vi "Top Level.vi"() -> ()   [LabVIEW 2018]
panel:
  in  "Frame Control":enum32{"0", "1", "2", "3", "4", "5", "6"}(tab)
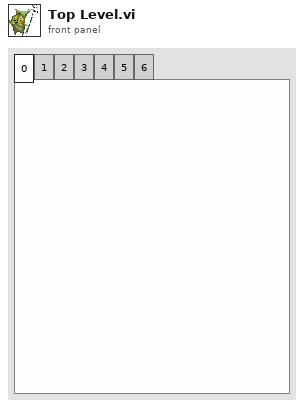
[diagram p1: front panel]
types:
  T1 = enum16{"Get_Item", "Yahaha!", "Korok_Pop", "Korok_Solve"}
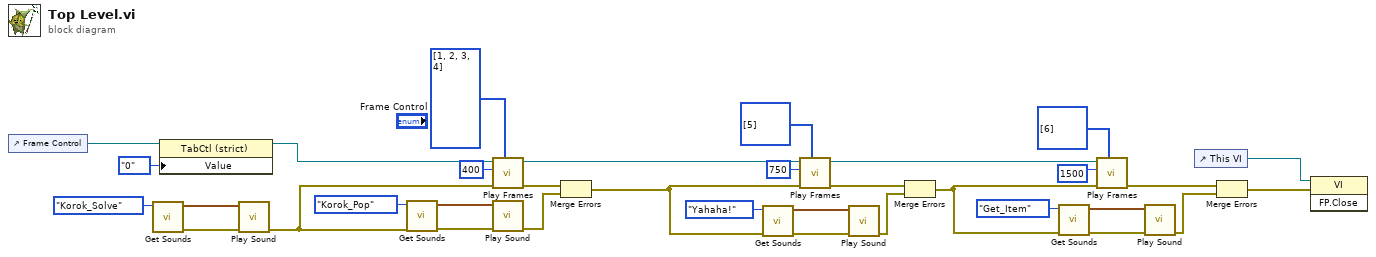
[diagram p0: block diagram]
diagram:
  n1 = control-ref of="Frame Control"() -> (w7:refnum<vi>)
  n2 = call "Get Sounds.vi"("Sound"=T1."Korok_Solve") -> ("error out"=w12:errorcluster, "Sound Out"=w11:waveform(dbl))  [unwired: 9 in]
  n3 = property class="TabCtl (strict)"(reference=w7, "Value"=enum32{"0", "1", "2", "3", "4", "5", "6"}."0") -> (reference out=w5:refnum<vi>)  [unwired: 1 in, 1 out]
  n4 = call "Play Sound.vi"("error in (no error)"=w12, "Sound"=w11) -> ("error out"=w9:errorcluster)  [unwired: 9 in]
  n5 = call "Get Sounds.vi"("error in (no error)"=w9, "Sound"=T1."Korok_Pop") -> ("error out"=w31:errorcluster, "Sound Out"=w32:waveform(dbl))  [unwired: 8 in]
  n6 = call "Play Frames.vi"("Frames (I:0)"=u32[] [1, 2, 3, 4], "error in (no error)"=w9, "Delay per Frame"=u32 400, "Frame Control Ref In"=w5) -> ("error out"=w30:errorcluster, "Frame Control Ref Out"=w27:refnum<vi>)  [unwired: 6 in]
  n7 = call "Play Sound.vi"("error in (no error)"=w31, "Sound"=w32) -> ("error out"=w29:errorcluster)  [unwired: 9 in]
  n8 = Merge Errors(w30, w29) -> (w13:errorcluster)
  n9 = call "Get Sounds.vi"("error in (no error)"=w13, "Sound"=T1."Yahaha!") -> ("error out"=w25:errorcluster, "Sound Out"=w24:waveform(dbl))  [unwired: 8 in]
  n10 = call "Play Frames.vi"("Frames (I:0)"=u32[] [5], "error in (no error)"=w13, "Delay per Frame"=u32 750, "Frame Control Ref In"=w27) -> ("error out"=w22:errorcluster, "Frame Control Ref Out"=w14:refnum<vi>)  [unwired: 6 in]
  n11 = call "Play Sound.vi"("error in (no error)"=w25, "Sound"=w24) -> ("error out"=w21:errorcluster)  [unwired: 9 in]
  n12 = Merge Errors(w22, w21) -> (w16:errorcluster)
  n13 = call "Get Sounds.vi"("error in (no error)"=w16, "Sound"=T1."Get_Item") -> ("error out"=w15:errorcluster, "Sound Out"=w17:waveform(dbl))  [unwired: 8 in]
  n14 = call "Play Frames.vi"("Frames (I:0)"=u32[] [6], "error in (no error)"=w16, "Delay per Frame"=u32 1500, "Frame Control Ref In"=w14) -> ("error out"=w3:errorcluster)  [unwired: 6 in, 1 out]
  n15 = call "Play Sound.vi"("error in (no error)"=w15, "Sound"=w17) -> ("error out"=w1:errorcluster)  [unwired: 9 in]
  n16 = control-ref of="This VI"() -> (w4:refnum<vi>)
  n17 = Merge Errors(w3, w1) -> (w2:errorcluster)
  n18 = invoke class="VI" method="FP.Close"(reference=w4, error in=w2) -> ()  [unwired: 1 in, 3 out]
